vi "探测器列表-更新累积剂量.vi"(6 "元素名[]-探测器信息":string[](array[string]), 7 "table名-探测器列表":string, 8 "error in (no error)":errorcluster, 9 "探测器信息":T2, 11 "数据库引用":T1) -> (0 "error out":errorcluster, 3 "connection reference out":T1)   [LabVIEW 2016]
doc: "只需传入 网络地址 和 累积剂量值 即可 , 其他元素可以空着 ."
uses:
  <vilib>/addons/database/Connection.llb/Conn ObjectReference.ctl
  <vilib>/addons/database/NI_Database_API.lvlib
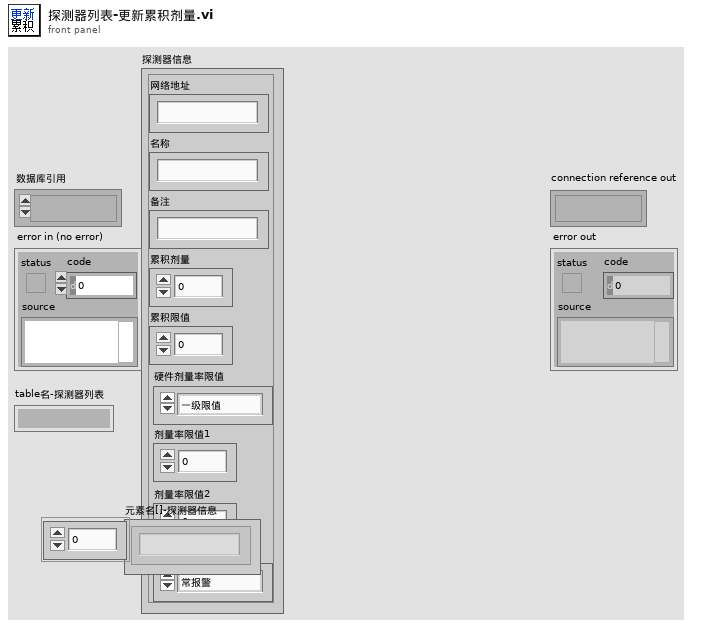
[diagram p1: front panel]
types:
  T1 = typedef "NI_Database_API.lvlib/Conn ObjectReference.ctl" = refnum<k1>
  T2 = typedef "探测器信息.ctl" = cluster{"网络地址":string, "名称":string, "备注":string, "累积剂量":dbl, "累积限值":dbl, "硬件剂量率限值":T3, "剂量率限值1":dbl, "剂量率限值2":dbl, "报警方式":T4}
  T3 = typedef "探头剂量率限值选择.ctl" = enum16{"一级限值", "二级限值"}
  T4 = typedef "报警方式选择.ctl" = enum16{"常报警", "自动静音", "手动静音"}
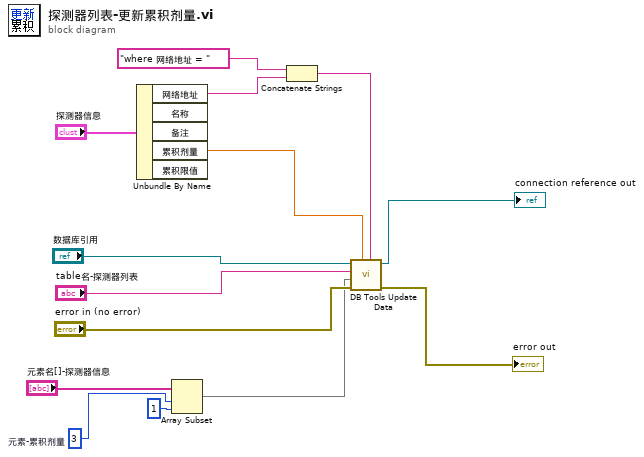
[diagram p0: block diagram]
diagram:
  w4 = 3  # 元素-累积剂量
  n1 = Unbundle By Name("探测器信息") -> ("网络地址"=w8:string, "累积剂量"=w1:dbl)  [unwired: 3 out]
  n2 = Array Subset(array="元素名[]-探测器信息", index=w4, length=1 ("长度")) -> (w2:string[])
  n3 = Concatenate Strings("where 网络地址 = " ("字符串"), w8) -> (w7:string)
  n4 = call <vilib>:"DB Tools Update Data.vi"("condition"=w7, "data"=w1, "error in (no error)"="error in (no error)", "columns"=w2, "table"="table名-探测器列表", "connection reference"="数据库引用") -> ("error out"=→"error out":errorcluster, "connection reference out"=→"connection reference out":T1)  [unwired: 4 in]
